vi "Main.vi"(8 "error in (no error)":errorcluster, 11 "Input Process in":refnum<class "Input Process.lvclass">) -> (0 "error out":errorcluster, 3 "Input Process out":refnum<class "Input Process.lvclass">)   [LabVIEW 2019, in "TimingDRV Engine.lvlib" / "Input Process.lvclass"]
uses:
  Input Process.lvclass
  Parent Classes/CD_Process/CD_Process.lvclass
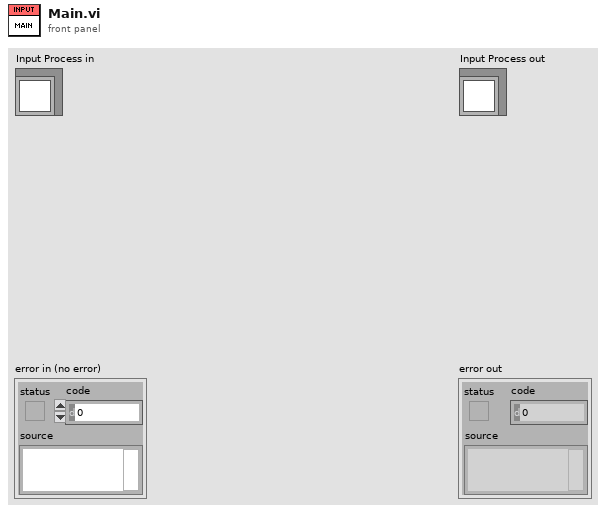
[diagram p1: front panel]
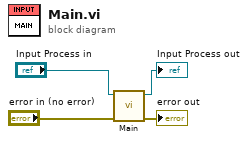
[diagram p0: block diagram]
diagram:
  n1 = call-parent "Main.vi"("error in (no error)"="error in (no error)", "CD_Process in"="Input Process in") -> ("error out"=→"error out":errorcluster, "CD_Process out"=→"Input Process out":refnum<class "Input Process.lvclass">)  [unwired: 8 in]
